vi "BL_GetVolumeSerialNumber.vi"(8 "error in (no error)":errorcluster, 11 "Potentiostat Galvanostat in":refnum<class "Potentiostat Galvanostat.lvclass">) -> (0 "error out":errorcluster, 2 "Serial Number":u32, 3 "Potentiostat Galvanostat out":refnum<class "Potentiostat Galvanostat.lvclass">)   [LabVIEW 2018, in "Potentiostat Galvanostat.lvclass"]
doc: "This function returns volume serial number.\n \nNote:\nThe serial number of a (logical) drive is generated every time a drive is formatted. When Windows formats a drive, a drive's serial number gets calculated using the current date and time and is stored in the drive's boot sector. The odds of two disks getting the same number are virtually nil on the same machine."
uses:
  Potentiostat Galvanostat.lvclass
  Potentiostat Galvanostat.lvclass/Potentiostat Galvanostat.ctl
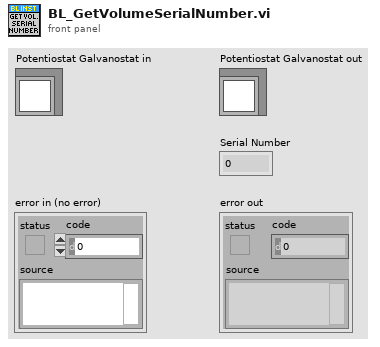
[diagram p1: front panel]
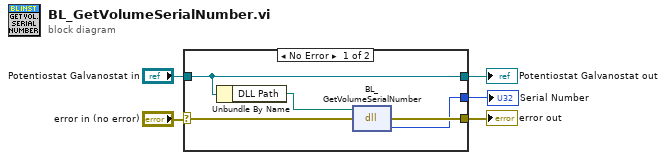
[diagram p0: block diagram]
diagram:
  n1 = case shown="No Error" "error in (no error)" {
    selector: "error in (no error)" -> [w8 w12]
    tunnel: [w7 w12] -> w4
    tunnel: [w10 w11] -> w2
    tunnel: "Potentiostat Galvanostat in" -> [w10 w11]
    tunnel: [w6 _] -> w1
    frame No Error {
      n2 = Unbundle By Name(w10) -> ("DLL Path"=w9:path)
      n3 = dll-call lib="C:/Projects/LabVIEW/BioLogic Instrument Driver/libs/EC-Lab Development Package/EClib.*" fn="BL_GetVolumeSerialNumber"(path in=w9, error in=w8) -> (error out=w7:errorcluster, "Serial Number"=w6:u32)  [unwired: 1 in, 1 out]
    }
    frame Error {
    }
  }
  "error out" <- w4
  "Potentiostat Galvanostat out" <- w2
  "Serial Number" <- w1
